vi "CRYStimulus Global.vi"() -> ()   [LabVIEW 2013]
uses:
  Typedef Control/CRYStimulus Cluster.ctl
panel:
  in  "ISO R80 series":dbl[](array[numeric])=[1.0, 1.0299999713897705, 1.059999942779541, 1.090000033378601, 1.1200000047683716, 1.149999976158142, 1.1799999475479126, 1.2200000286102295, 1.25, 1.2799999713897705, 1.3200000524520874, 1.3600000143051147, 1.399999976158142, 1.4500000476837158, 1.5, 1.5499999523162842, 1.600000023841858, 1.649999976158142, 1.7000000476837158, 1.75, 1.7999999523162842, 1.850000023841858, 1.899999976158142, 1.9500000476837158, 2.0, 2.059999942779541, 2.119999885559082, 2.180000066757202, 2.240000009536743, 2.299999952316284, 2.359999895095825, 2.430000066757202, 2.5, 2.5799999237060547, 2.6500000953674316, 2.7200000286102295, 2.799999952316284, 2.9000000953674316, 3.0, 3.069999933242798, 3.1500000953674316, 3.25, 3.3499999046325684, 3.450000047683716, 3.549999952316284, 3.6500000953674316, 3.75, 3.869999885559082, 4.0, 4.119999885559082, 4.25, 4.369999885559082, 4.5, 4.619999885559082, 4.75, 4.869999885559082, 5.0, 5.150000095367432, 5.300000190734863, 5.449999809265137, 5.599999904632568, 5.800000190734863, 6.0, 6.150000095367432, 6.300000190734863, 6.5, 6.699999809265137, 6.900000095367432, 7.099999904632568, 7.300000190734863, 7.5, 7.75, 8.0, 8.25, 8.5, 8.75, 9.0, 9.25, 9.5, 9.75, 10.0, 10.300000190734863, 10.600000381469727, 10.899999618530273, 11.199999809265137, 11.5, 11.800000190734863, 12.199999809265137, 12.5, 12.800000190734863, 13.199999809265137, 13.600000381469727, 14.0, 14.5, 15.0, 15.5, 16.0, 16.5, 17.0, 17.5, 18.0, 18.5, 19.0, 19.5, 20.0, 20.600000381469727, 21.200000762939453, 21.799999237060547, 22.399999618530273, 23.0, 23.600000381469727, 24.299999237060547, 25.0, 25.799999237060547, 26.5, 27.200000762939453, 28.0, 29.0, 30.0, 30.700000762939453, 31.5, 32.5, 33.5, 34.5, 35.5, 36.5, 37.5, 38.70000076293945, 40.0, 41.20000076293945, 42.5, 43.70000076293945, 45.0, 46.20000076293945, 47.5, 48.70000076293945, 50.0, 51.5, 53.0, 54.5, 56.0, 58.0, 60.0, 61.5, 63.0, 65.0, 67.0, 69.0, 71.0, 73.0, 75.0, 77.5, 80.0, 82.5, 85.0, 87.5, 90.0, 92.5, 95.0, 97.5, 100.0, 103.0, 106.0, 109.0, 112.0, 115.0, 118.0, 122.0, 125.0, 128.0, 132.0, 136.0, 140.0, 145.0, 150.0, 155.0, 160.0, 165.0, 170.0, 175.0, 180.0, 185.0, 190.0, 195.0, 200.0, 206.0, 212.0, 218.0, 224.0, 230.0, 236.0, 243.0, 250.0, 258.0, 265.0, 272.0, 280.0, 290.0, 300.0, 307.0, 315.0, 325.0, 335.0, 345.0, 355.0, 365.0, 375.0, 387.0, 400.0, 412.0, 425.0, 437.0, 450.0, 462.0, 475.0, 487.0, 500.0, 515.0, 530.0, 545.0, 560.0, 580.0, 600.0, 615.0, 630.0, 650.0, 670.0, 690.0, 710.0, 730.0, 750.0, 775.0, 800.0, 825.0, 850.0, 875.0, 900.0, 925.0, 950.0, 975.0, 1000.0, 1030.0, 1060.0, 1090.0, 1120.0, 1150.0, 1180.0, 1220.0, 1250.0, 1280.0, 1320.0, 1360.0, 1400.0, 1450.0, 1500.0, 1550.0, 1600.0, 1650.0, 1700.0, 1750.0, 1800.0, 1850.0, 1900.0, 1950.0, 2000.0, 2060.0, 2120.0, 2180.0, 2240.0, 2300.0, 2360.0, 2430.0, 2500.0, 2580.0, 2650.0, 2720.0, 2800.0, 2900.0, 3000.0, 3070.0, 3150.0, 3250.0, 3350.0, 3450.0, 3550.0, 3650.0, 3750.0, 3870.0, 4000.0, 4120.0, 4250.0, 4370.0, 4500.0, 4620.0, 4750.0, 4870.0, 5000.0, 5150.0, 5300.0, 5450.0, 5600.0, 5800.0, 6000.0, 6150.0, 6300.0, 6500.0, 6700.0, 6900.0, 7100.0, 7300.0, 7500.0, 7750.0, 8000.0, 8250.0, 8500.0, 8750.0, 9000.0, 9250.0, 9500.0, 9750.0, 10000.0, 10300.0, 10600.0, 10900.0, 11200.0, 11500.0, 11800.0, 12200.0, 12500.0, 12800.0, 13200.0, 13600.0, 14000.0, 14500.0, 15000.0, 15500.0, 16000.0, 16500.0, 17000.0, 17500.0, 18000.0, 18500.0, 19000.0, 19500.0, 20000.0, 20600.0, 21200.0, 21800.0, 22400.0, 23000.0, 23600.0, 24300.0, 25000.0, 25800.0, 26500.0, 27200.0, 28000.0, 29000.0, 30000.0, 30700.0, 31500.0, 32500.0, 33500.0, 34500.0, 35500.0, 36500.0, 37500.0, 38700.0, 40000.0, 41200.0, 42500.0, 43700.0, 45000.0, 46200.0, 47500.0, 48700.0, 50000.0, 51500.0, 53000.0, 54500.0, 56000.0, 58000.0, 60000.0, 61500.0, 63000.0, 65000.0, 67000.0, 69000.0, 71000.0, 73000.0, 75000.0, 77500.0, 80000.0] format="%.2f"
  in  "OK flg":bool
  out "Flatten Element Out":string
  in  "List Index":i32
  in  "End flg":bool
  in  "Stimulus Cluster":T1={"StimulusType"="", "UseMLValArray"=[], "ML_axisArray"=[], "MLValLevelNameArray"=[], "Level(U)Array"=[1.0, 0.0, 0.0, 0.0, 0.0, 0.0, 0.26], "Start(Stop)FreqArray"=[20000.0, 20.0], "Start(Stop)AmpArray"=[0.5, 1.0], "StepResolutionArray"=[], "Unit_Array"=[], "DegValArray"=[], "DegUnitArray"=[], "Steps1"=19, "Cycle/step1(#)"=20, "Time/step1(s)"=0.01, "Transition1"=0.0, "SweepRate2"=1.0, "Freq3(Hz)"=0.0, "Steps3(#)"=19.0, "Cycles3(#)"=12, "StepSize3"=0.0, "wave time"="", "RMS_Value4"=0.0, "Peak_Value4"=0.0, "WavePath4"="", "RMS_unit4"="", "Peak_unit4"="", "wave Info"="", "dc_ctrl5_1"=0, "dc_ctrl5_2"=0, "dc_polar5"=0, "Max.Current"=0, "Steps5(#)"=19, "Time/Step5"=0.05, "Level5"=0.0, "StepsSize5Val"=0.0, "StepSize5Unit"="", "SweepType"=0, "Fixed/Ratio6"=0, "Transition6"=0.0, "Steps6(#)"=19.0, "Cycle/Steps6(#)"=12, "Time/Steps6(s)"=0.0, "Freq6(Hz)"=0.0, "Difference6(Hz)"=0.0, "Ratio6"="", "NoiseType7"=0, "Duration7(s)"=1.0, "MinFreq7(Hz)"=20000.0, "MaxFreq7(Hz)"=20.0, "MinFreq8(Hz)"=20000.0, "MaxFreq8(Hz)"=20.0, "FreqRounding8"=FALSE, "Duration8(s)"=1.0, "Tones8"=0.0, "RoundingVal8"=0.0, "ApplyEQ"=FALSE, "Duration(s)"=0.0, "CustomStimulusName "="", "Flatten Element Array"=[], "sine waves"=[], "Channel Out"=0, "RatioVal6"=0.0, "TabCtrl6"=enum."Master Tone", "Signal Type Name"="", "Help"="", "Channel Sel"=0, "V on DUT"=FALSE, "Output Imp"=6300.0, "Nominal Imp"=100.0} {"Nominal Imp" format="%.2p"; "Output Imp" format="%.2p"; "sine waves"."cycles" format="%.2f"; "sine waves"."ampl" format="%.2f"; "sine waves"."freq" format="%.2f"}
  in  "Old Curve Name":string
  in  "Stimulus Vi Ref":refnum<vi>
  in  "Flatten Element":string
  out "Flatten Element Stimulus SetupCluster":T2
  # "(1,2,3,4,6_1,6_2,7,8)"
  # "(1,2,3,4,6_1,6_2,7,8)"
  # "(1,2,3,4,6_1,6_2,7,8)"
  # "(1,2,4,6_1,6_2,7,8)"
  # "(1,2,6)"
  # "(3,5)"
  # "(1,6,8)"
  # "(1,2,4,6_1,6_2,7,8)"
  # "(1,2,3,4,6_1,6_2,7,8)"
  # "(1,2,3,4,6_1,6_2,7,8)"
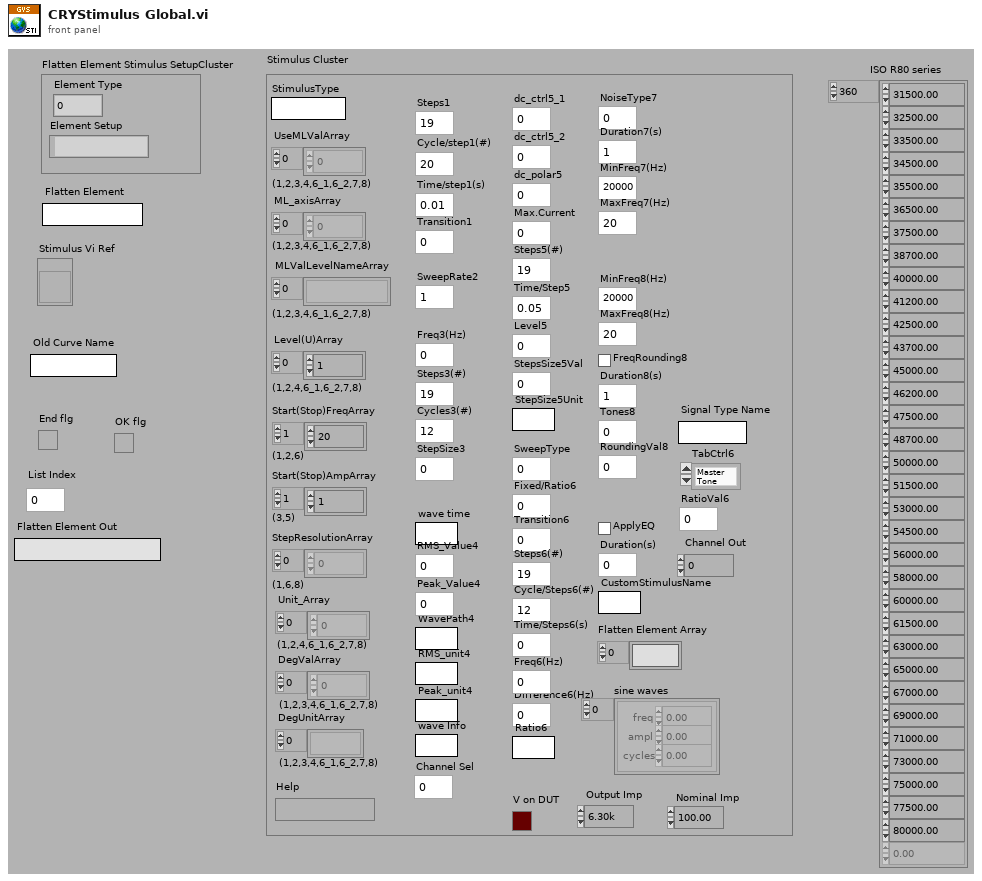
[diagram p1: front panel]
types:
  T1 = typedef "CRYStimulus Cluster.ctl" = cluster{"StimulusType":string, "UseMLValArray":u16[], "ML_axisArray":u16[], "MLValLevelNameArray":string[], "Level(U)Array":dbl[], "Start(Stop)FreqArray":dbl[], "Start(Stop)AmpArray":dbl[], "StepResolutionArray":u16[], "Unit_Array":u16[], "DegValArray":dbl[], "DegUnitArray":string[], "Steps1":i32, "Cycle/step1(#)":u32, "Time/step1(s)":dbl, "Transition1":dbl, "SweepRate2":dbl, "Freq3(Hz)":dbl, "Steps3(#)":dbl, "Cycles3(#)":u32, "StepSize3":dbl, "wave time":string, "RMS_Value4":dbl, "Peak_Value4":dbl, "WavePath4":string, "RMS_unit4":string, "Peak_unit4":string, "wave Info":string, "dc_ctrl5_1":u16, "dc_ctrl5_2":u16, "dc_polar5":u16, "Max.Current":u16, "Steps5(#)":u32, "Time/Step5":dbl, "Level5":dbl, "StepsSize5Val":dbl, "StepSize5Unit":string, "SweepType":u16, "Fixed/Ratio6":u16, "Transition6":dbl, "Steps6(#)":dbl, "Cycle/Steps6(#)":u32, "Time/Steps6(s)":dbl, "Freq6(Hz)":dbl, "Difference6(Hz)":dbl, "Ratio6":string, "NoiseType7":u16, "Duration7(s)":dbl, "MinFreq7(Hz)":dbl, "MaxFreq7(Hz)":dbl, "MinFreq8(Hz)":dbl, "MaxFreq8(Hz)":dbl, "FreqRounding8":bool, "Duration8(s)":dbl, "Tones8":dbl, "RoundingVal8":dbl, "ApplyEQ":bool, "Duration(s)":dbl, "CustomStimulusName ":string, "Flatten Element Array":string[], "sine waves":cluster{"freq":dbl, "ampl":dbl, "cycles":dbl}[], "Channel Out":i32, "RatioVal6":dbl, "TabCtrl6":enum32{"Master Tone", "Slave Tone"}, "Signal Type Name":string, "Help":string, "Channel Sel":u16, "V on DUT":bool, "Output Imp":dbl, "Nominal Imp":dbl}
  T2 = cluster{"Element Type":u32, "Element Setup":string}
diagram:
